vi "Get Flattened Image.vi"(8 "error in":errorcluster, 11 "lv_icon.lvlib:Icon.lvclass in":refnum<class "Icon.lvclass">) -> (0 "error out":errorcluster, 1 "BW Image":T1, 2 "Color Image":T1, 3 "lv_icon.lvlib:Icon.lvclass out":refnum<class "Icon.lvclass">)   [LabVIEW 2020, in "LabVIEW Icon API.lvlib"]
doc: "Takes the information that is stored in the Icon class and creates the corresponding Color and BW icon."
uses:
  LabVIEW Icon API.lvlib
  lv_icon/Classes/Icon/Icon.lvclass
  lv_icon/Classes/Icon Framework/Icon Framework.lvclass
  lv_icon/lv_icon.lvlib
  <vilib>/picture/picture.llb/imagedata.ctl
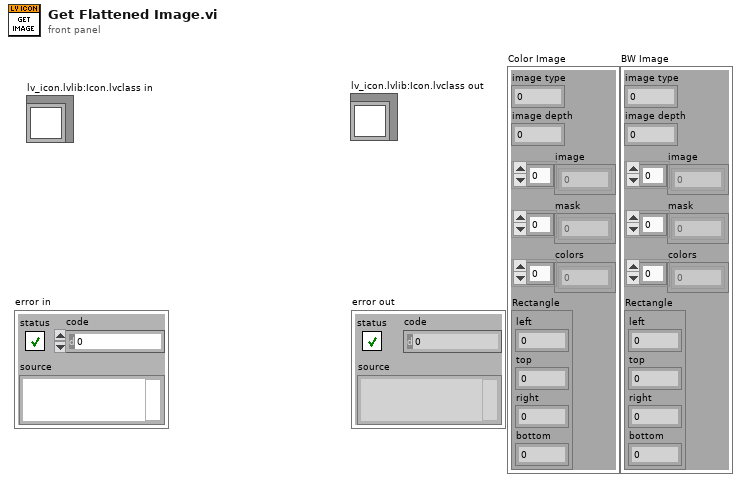
[diagram p1: front panel]
types:
  T1 = typedef "imagedata.ctl" = cluster{"image type":i32, "image depth":i32, "image":u8[], "mask":u8[], "colors":u32[], "Rectangle":cluster{"left":i16, "top":i16, "right":i16, "bottom":i16}}
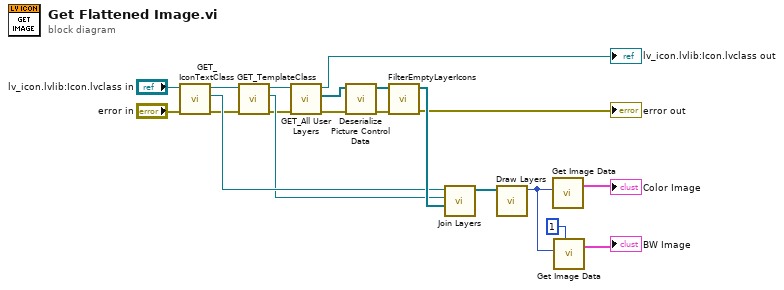
[diagram p0: block diagram]
diagram:
  n1 = call-dynamic "GET_IconTextClass.vi"("error in (no error)"="error in", "Icon.lvclass in"="lv_icon.lvlib:Icon.lvclass in") -> ("error out"=w8:errorcluster, "Icon Framework.lvclass"=w11:refnum<class "Icon Framework.lvclass">, "Icon.lvclass out"=w15:refnum<class "Icon.lvclass">)  [unwired: 7 out]
  n2 = call-dynamic "GET_TemplateClass.vi"("error in (no error)"=w8, "Icon.lvclass in"=w15) -> ("error out"=w9:errorcluster, "Icon Framework.lvclass"=w10:refnum<class "Icon Framework.lvclass">, "Icon.lvclass out"=w16:refnum<class "Icon.lvclass">)  [unwired: 7 in]
  n3 = call-dynamic "GET_All User Layers.vi"("error in (no error)"=w9, "Icon.lvclass in"=w16) -> ("error out"=w17:errorcluster, "User Layer"=w18:refnum<class "Layer.lvclass">[], "Icon.lvclass out"=→"lv_icon.lvlib:Icon.lvclass out":refnum<class "Icon.lvclass">)  [unwired: 7 in]
  n4 = call "Deserialize Picture Control Data.vi"("error in (no error)"=w17, "Layers in"=w18) -> ("error out"=w20:errorcluster, "Layers out"=w19:refnum<class "Layer.lvclass">[])  [unwired: 8 out]
  n5 = call "FilterEmptyLayerIcons.vi"("error in (no error)"=w20, "Layers"=w19) -> ("error out"=→"error out":errorcluster, "Layers out"=w12:refnum<class "Layer.lvclass">[])  [unwired: 8 out]
  n6 = call "Join Layers.vi"("User Layers"=w12, "Template"=w10, "Icon Text"=w11) -> ("Layer out"=w14:refnum<class "Layer.lvclass">[])  [unwired: 3 in, 5 out]
  n7 = call "Draw Layers.vi"("Layers"=w14) -> ("Picture"=w13:picture)  [unwired: 4 in, 6 out]
  n8 = call "Get Image Data.vi"("Pic In"=w13) -> ("image data out"=→"Color Image":T1)  [unwired: 2 in, 8 out]
  n9 = call "Get Image Data.vi"("depth (24)"=1 ("depth"), "Pic In"=w13) -> ("image data out"=→"BW Image":T1)  [unwired: 2 in, 7 out]
